vi "SDSU_MemLocDefs.vi"(8 "error in (no error)":errorcluster, 9 "action":enum16{"read from file", "find", "clear"}(ring), 10 "name":string, 11 "translations path":path=path "/home/sensei/fpas/_lskipper/config/DETECTOR/command_translations.cfg") -> (1 "found":bool, 2 "location":string, 3 "memlocs":T1[](array[typedef]))   [LabVIEW 2016]
uses:
  SDSU_MemLocStruct.ctl
  <vilib>/Utility/config.llb/Read Key (String).vi
  <vilib>/Utility/config.llb/NI_LVConfig.lvlib
panel:
  in  "ele":T1
  out "translations path 2":path=path "/home/bonati/PAN/Modules/MNSN/private/c/test/command_translations.cfg"
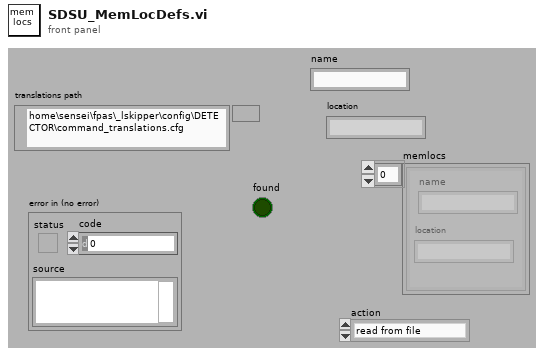
[diagram p1: front panel]
types:
  T1 = typedef "SDSU_MemLocStruct.ctl" = cluster{"name":string, "location":string}
  T2 = typedef "NI_LVConfig.lvlib/Config Data RefNum.ctl" = refnum<k1>
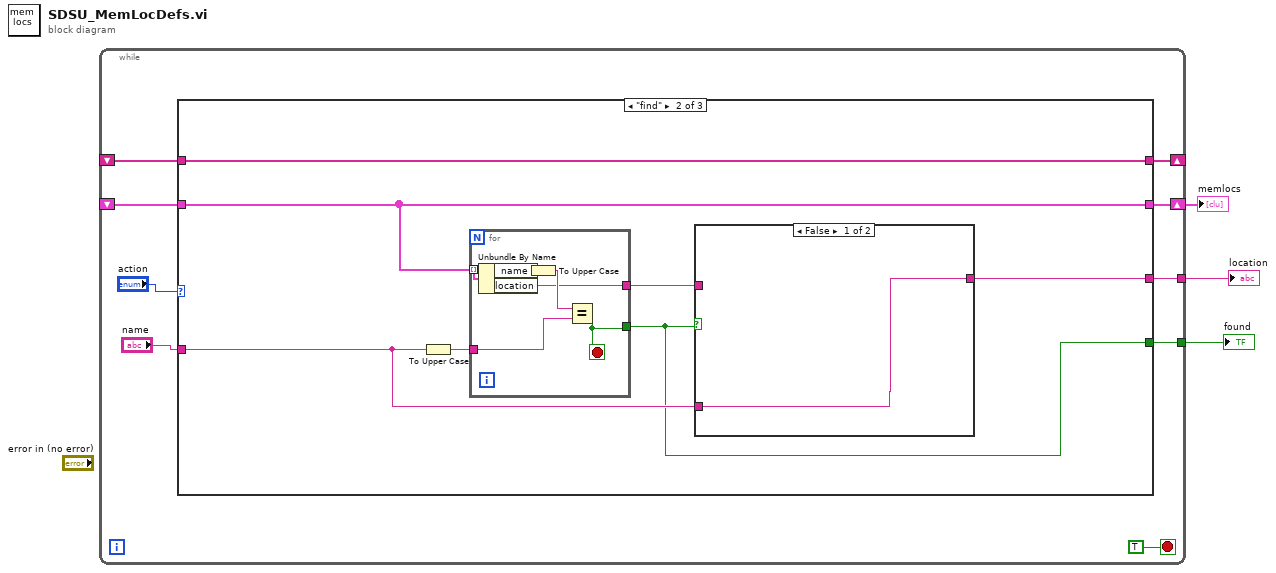
[diagram p0: block diagram]
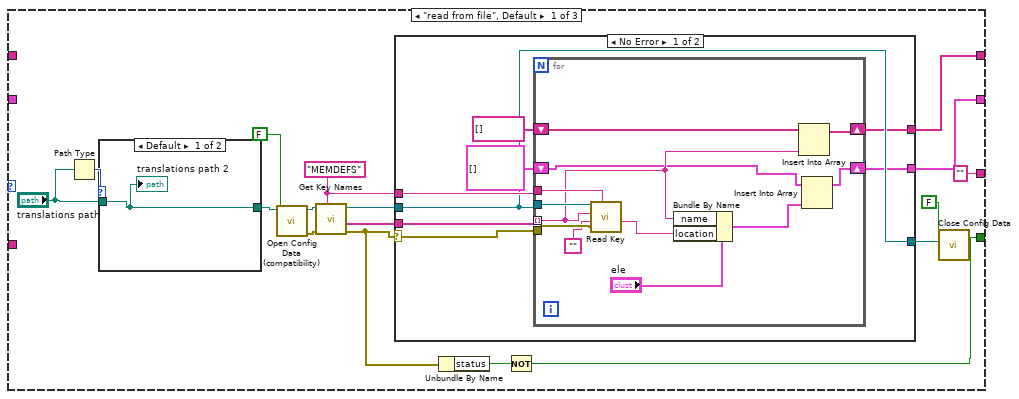
[diagram p2: hidden frame]
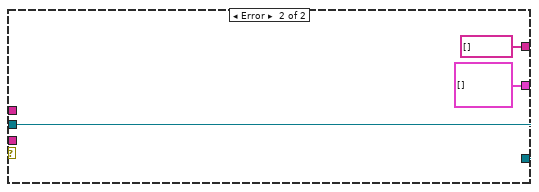
[diagram p3: hidden frame]
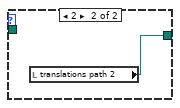
[diagram p4: hidden frame]
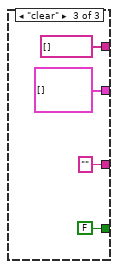
[diagram p6: hidden frame]
diagram:
  n1 = while {
    shift-right: [w9] -> w3
    shift-left: _ -> [w7]
    shift-right: [w10] -> _
    shift-left: _ -> [w8]
    tunnel: [w5] -> w2
    tunnel: [w4] -> w1
    stop <- TRUE stop-if-true
    n2 = case shown="\"find\"" "action" {
      tunnel: [w18 w61 string[] []] -> w10
      tunnel: [w17 w60 T1[] []] -> w9
      tunnel: w8 -> [_ w61 _]
      tunnel: w7 -> [_ w60 _]
      tunnel: "name" -> [_ w56 _]
      tunnel: ["" ("location") w57 "" ("location")] -> w5
      tunnel: [w13 w55 FALSE] -> w4
      frame "read from file", Default {
        w25 = "MEMDEFS" ("section")
        n3 = Path Type(1:"translations path") -> (0:w24:i16)
        n4 = case shown="Default" w24 {
          tunnel: "translations path" -> [w53 _]
          tunnel: [w53 w54] -> w22
          frame Default {
            "translations path 2" <- w53
          }
          frame 2 {
            n5 = local read "translations path 2"() -> (w54:path)
          }
        }
        n6 = call <vilib>:"Open Config Data (compatibility).vi"("create file if necessary (T)"=FALSE, "configuration file path"=w22) -> ("error out"=w29:errorcluster, "refnum"=w28:T2)  [unwired: 7 in, 1 out]
        n7 = call <vilib>:"Get Key Names.vi"("section"=w25, "error in (no error)"=w29, "refnum"=w28) -> ("error out"=w15:errorcluster, "key names"=w27:string[], "refnum out"=w26:T2)  [unwired: 6 out]
        n8 = case shown="No Error" w15 {
          selector: w15 -> [w33 _]
          tunnel: w27 -> [w37 _]
          tunnel: w26 -> [w35 w52]
          tunnel: w25 -> [w36 _]
          tunnel: [w35 w52] -> w21
          tunnel: [w31 string[] []] -> w18
          tunnel: [w30 T1[] []] -> w17
          frame No Error {
            n9 = for {
              tunnel: w37 -> [w42] mode=indexing
              tunnel: w35 -> [w49]
              tunnel: w33 -> [w48]
              tunnel: w36 -> [w47]
              shift-right: [w40] -> w31
              shift-left: string[] [] -> [w41]
              shift-right: [w39] -> w30
              shift-left: T1[] [] -> [w38]
              n10 = call-poly <vilib>:"Read Key.vi"("section"=w47, "error in (no error)"=w48, "default value"="", "key"=w42, "refnum"=w49) -> ("value"=w44:string)  [unwired: 1 in, 5 out]
              n11 = Bundle By Name(cluster="ele", "name"=w42, "location"=w44) -> (w43:T1)
              n12 = Insert Into Array(array=w41, new element=w42) -> (w40:string[])  [unwired: 1 in]
              n13 = Insert Into Array(array=w38, new element=w43) -> (w39:T1[])  [unwired: 1 in]
            }
          }
          frame Error {
          }
        }
        n14 = Unbundle By Name(w15) -> ("status"=w14:bool)
        n15 = Not(x=w14) -> (.not. x?=w13:bool)
        n16 = call <vilib>:"Close Config Data.vi"("write file if changed (T)"=FALSE ("write configuration file? (T)"), "refnum"=w21) -> ()  [unwired: 1 in, 9 out]
      }
      frame "find" {
        n17 = To Upper Case(1:w56) -> (0:w59:string)
        n18 = for {
          tunnel: w60 -> [w69] mode=indexing
          tunnel: w59 -> [w67]
          tunnel: [w65] -> w55
          tunnel: [w64] -> w58
          stop <- w65 stop-if-true
          n19 = Unbundle By Name(w69) -> ("name"=w68:string, "location"=w64:string)
          n20 = To Upper Case(1:w68) -> (0:w66:string)
          n21 = Equal?(x=w66, y=w67) -> (x = y?=w65:bool)
        }
        n22 = case shown="False" w55 {
          tunnel: w58 -> [_ w63]
          tunnel: [w62 w63] -> w57
          tunnel: w56 -> [w62 _]
          frame False {
          }
          frame True {
          }
        }
      }
      frame "clear" {
      }
    }
  }
  "memlocs" <- w3
  "found" <- w1
  "location" <- w2
